vi "WebCam.Disconnect.vi"(0 "Handle":i32, 11 "ErrorIn":errorcluster) -> (15 "ErrorOut":errorcluster)   [LabVIEW 2021]
uses:
  User32.WebCam_WM_Events.ctl
  User32.SendMessageA_num.vi
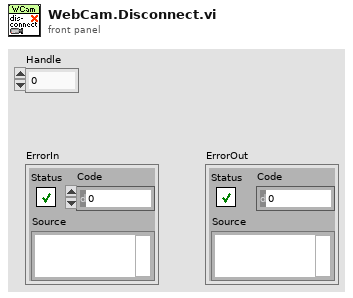
[diagram p1: front panel]
types:
  T1 = typedef "User32.WebCam_WM_Events.ctl" = i32
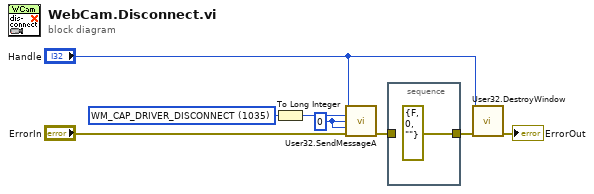
[diagram p0: block diagram]
diagram:
  w2 = T1 1035 items=["WM_CAP_DRIVER_CONNECT"=1034, "WM_CAP_DRIVER_DISCONNECT"=1035, "WM_CAP_EDIT_COPY"=1054, "WM_CAP_SEQUENCE"=1086, "WM_CAP_FILE_SAVEAS"=1047, "WM_CAP_SET_SCALE"=1077, "WM_CAP_SET_PREVIEWRATE"=1076, "WM_CAP_SET_PREVIEW"=1074, "WM_CAP_SET_OVERLAY"=1075, "WM_CAP_FILE_SAVEDIB"=1049] ("Ring")
  w3 = 0
  n1 = To Long Integer(number=w2) -> (32bit integer=w1:T1)
  n2 = call-poly "User32.SendMessageA.vi"("HWnd"="Handle", "Msg"=w1, "WParam"=w3, "LParam"=w3, "ErrorIn"="ErrorIn") -> ("ErrorOut"=w8:errorcluster)  [unwired: 9 in, 1 out]
  n3 = stacked-sequence {
    tunnel: [errorcluster {"status"=FALSE, "code"=0, "source"=""} ("error in (no error)")] -> w7
    tunnel: w8 -> [_]
    frame #0 {
    }
  }
  n4 = call "User32.DestroyWindow.vi"("HWnd"="Handle", "ErrorIn"=w7) -> ("ErrorOut"=→"ErrorOut":errorcluster)  [unwired: 13 in]
